vi "cast u64 to s-64-32.vi"(11 "aofxp":u64) -> (3 "fixedpoint_o":fxp<+/-,64,32>)   [LabVIEW 2020, in "fixedpoint-cast.lvlib"]
uses:
  fixedpoint-cast.lvlib
  <vilib>/rvi/IPIntegrationNode/IPINode_Typedef/niFpgaIPINodeSupportedFamilies.ctl
  <vilib>/rvi/IPIntegrationNode/IPINode_Utilities/niFpgaIPINodeSimCore.vi
  <vilib>/rvi/IPIntegrationNode/IPINode_Xnode/niFpgaIPINode.xnode
  fixedpoint_vhdl/src/cast_u64_to_s_dash_64_dash_32SimFiles/xsim.dir/u64_to_fixedpoint/xsimkF35A88E02AA440E4AED59715AE28C165.dll
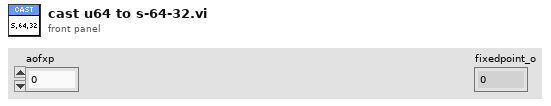
[diagram p1: front panel]
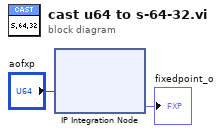
[diagram p0: block diagram]
diagram:
  n1 = xnode "IP Integration Node"("u64_i"="aofxp") -> ("fixedpoint_o"=→"fixedpoint_o":fxp<+/-,64,32>)
